vi "Save Waveform Chart history.vi"   [LabVIEW 2026, in "TALOS.lvlib" / "Father of all uServices.lvlib" / "Father of all uServices.lvclass"]
uses:
  Father of all uServices.lvclass
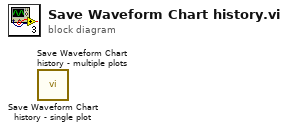
[diagram p0: block diagram]
diagram:
  n1 = call "Save Waveform Chart history - single plot.vi"() -> ()  [unwired: 10 in, 2 out]
  n2 = call "Save Waveform Chart history - multiple plots.vi"() -> ()  [unwired: 10 in, 2 out]
